vi "Register Variation.vi"() -> ()   [LabVIEW 2014]
uses:
  TypeDef/state.ctl
  TypeDef/Qmessage.ctl
  <vilib>/Utility/config.llb/Read Key (Path).vi
  <vilib>/Utility/file.llb/Read From Spreadsheet File (string).vi
  <vilib>/Utility/config.llb/Write Key (Path).vi
  <vilib>/Utility/config.llb/NI_LVConfig.lvlib
panel:
  in  "Help Button":bool
  in  "Run":bool
  in  "Initialize":bool
  out "Status bar":string
  in  "Register change":bool
  in  "Add comment":bool
  in  "View":bool
  in  "NV 31":string
  in  "NV 30":string
  in  "NV 29":string
  in  "NV 28":string
  in  "NV 27":string
  in  "NV 26":string
  in  "NV 25":string
  in  "NV 24":string
  in  "NV 23":string
  in  "NV 22":string
  in  "NV 21":string
  in  "NV 20":string
  in  "NV 19":string
  in  "NV 18":string
  in  "NV 17":string
  in  "NV 16":string
  in  "NV 15":string
  in  "NV 14":string
  in  "NV 13":string
  in  "NV 12":string
  in  "NV 11":string
  in  "NV 10":string
  in  "NV 9":string
  in  "NV 8":string
  in  "NV 7":string
  in  "NV 6":string
  in  "NV 5":string
  in  "NV 4":string
  in  "NV 3":string
  in  "NV 2":string
  in  "NV 1":string
  out "V 31":string
  out "V 30":string
  out "V 29":string
  out "V 28":string
  out "V 27":string
  out "V 26":string
  out "V 25":string
  out "V 24":string
  out "V 23":string
  out "V 22":string
  out "V 21":string
  out "V 20":string
  out "V 19":string
  out "V 18":string
  out "V 17":string
  out "V 16":string
  out "V 15":string
  out "V 14":string
  out "V 13":string
  out "V 12":string
  out "V 11":string
  out "V 10":string
  out "V 9":string
  out "V 8":string
  out "V 7":string
  out "V 6":string
  out "V 5":string
  out "V 4":string
  out "V 3":string
  out "V 2":string
  out "V 1":string
  in  "tdms path":path caption="Variation Registry (*.tdms)"
  in  "Config Path":path caption="Config Path (*.txt)"
  out "N 31":string
  out "N 30":string
  out "N 29":string
  out "N 28":string
  out "N 27":string
  out "N 26":string
  out "N 25":string
  out "N 24":string
  out "N 23":string
  out "N 22":string
  out "N 21":string
  out "N 20":string
  out "N 19":string
  out "N 18":string
  out "N 17":string
  out "N 16":string
  out "N 15":string
  out "N 14":string
  out "N 13":string
  out "N 12":string
  out "N 11":string
  out "N 10":string
  out "N 9":string
  out "N 8":string
  out "N 7":string
  out "N 6":string
  out "N 5":string
  out "N 4":string
  out "N 3":string
  out "N 2":string
  out "N 1":string
  in  "Exit":bool
  # "Change Register"
  # "Current Configuration"
  # "New Configuration"
  # "Component Name"
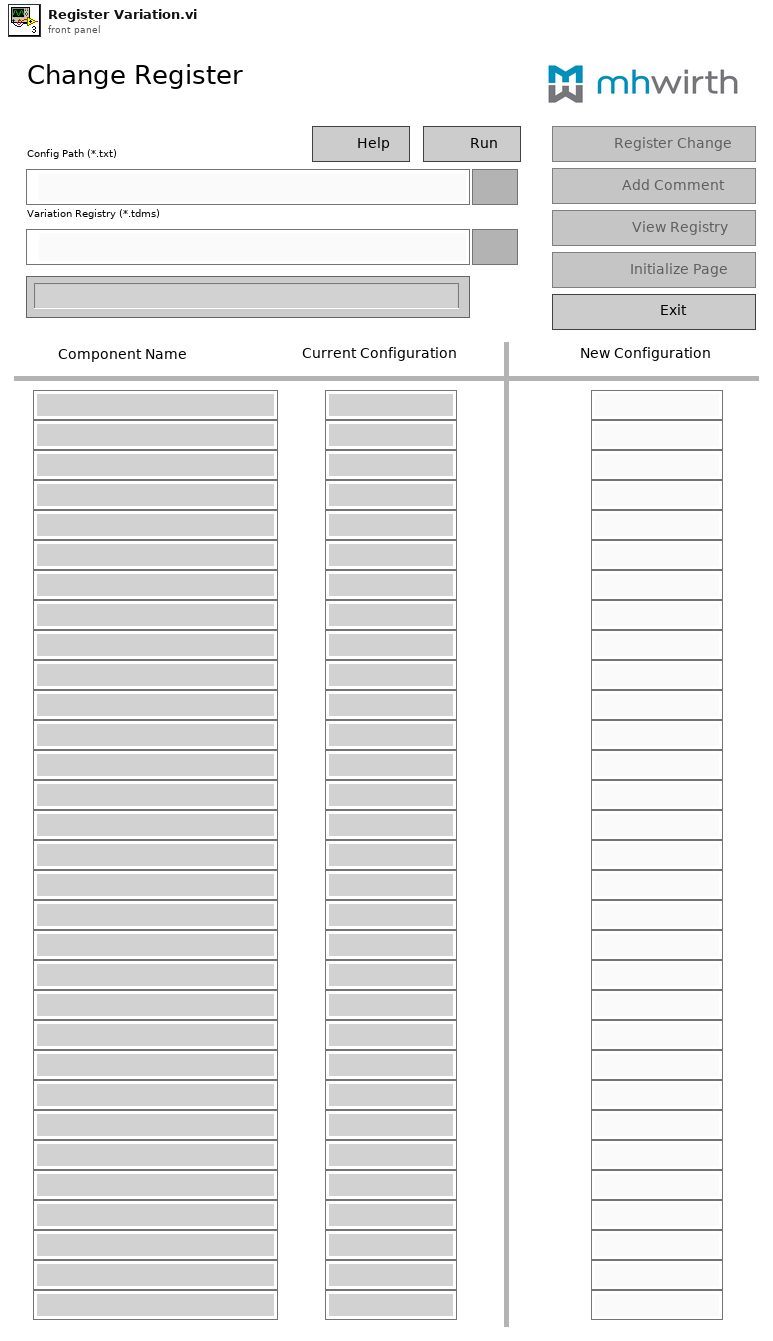
[diagram p1: front panel]
types:
  T1 = typedef "Qmessage.ctl" = cluster{"data":variant, "state":T2}
  T2 = typedef "state.ctl" = enum16{"Run", "Initialize 1", "Initialize 2", "Read config file", "Read TDMS", "Config file Error", "Idle", "Update Comp Names", "Update Current Versions", "Make new configuration", "Register Change", "View Registry", "Add Comment", "No New Update", "Check current versions", "Read ini file", "Write ini file", "Close"}
  T3 = enum32{"invalid app kind", "Development System", "Run Time System", "Student Edition", "Embedded LabVIEW", "Evaluation", "Custom"}
  T4 = cluster{"keys":refnum<vi>[], "Names":refnum<vi>[], "Current Versions":refnum<vi>[], "New Versions":refnum<vi>[]}
  T5 = enum8{"Enabled", "Disabled", "Disabled and Grayed Out"}
  T6 = typedef "NI_LVConfig.lvlib/Config Data RefNum.ctl" = refnum<k1>
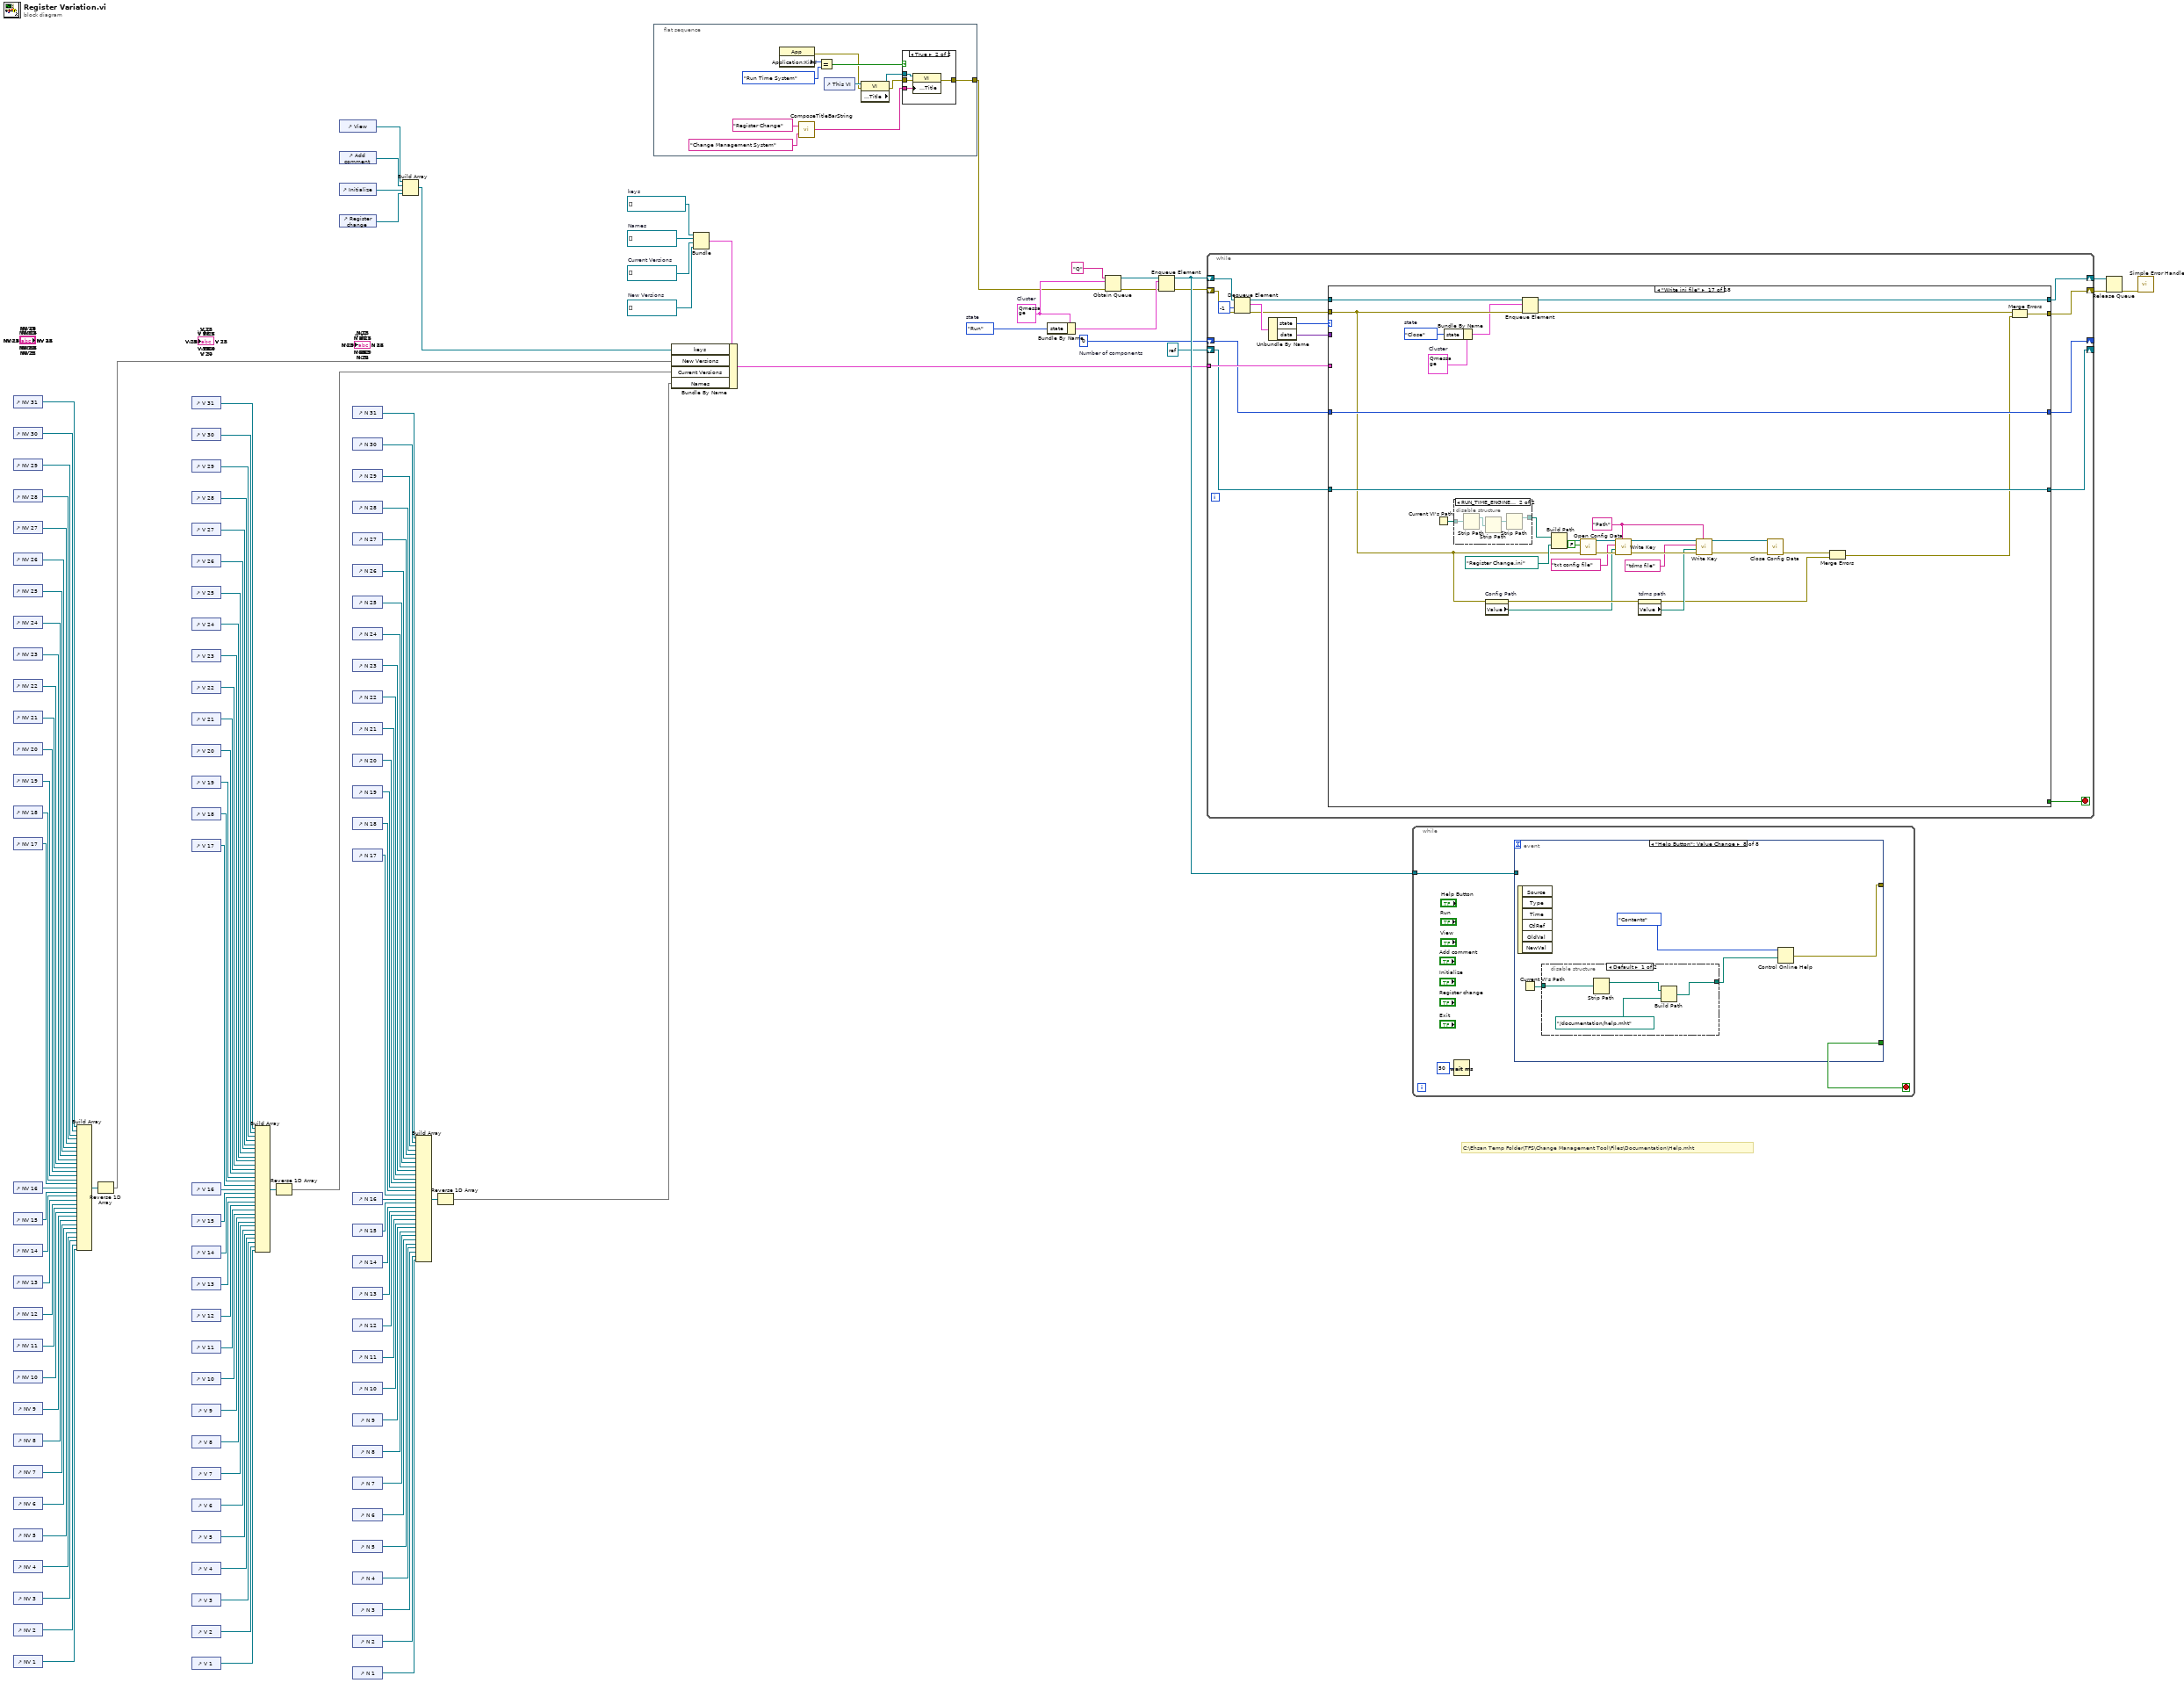
[diagram p0: block diagram]
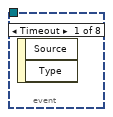
[diagram p3: hidden frame]
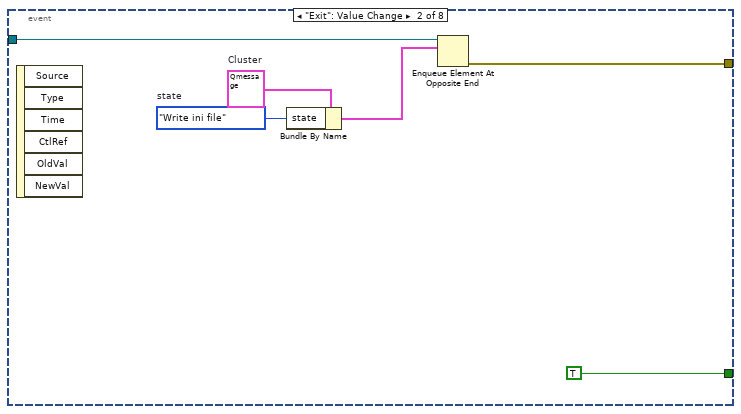
[diagram p4: hidden frame]
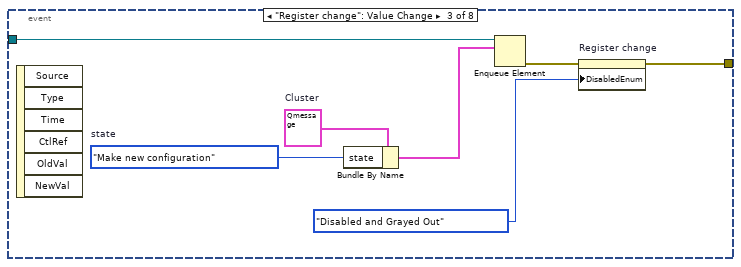
[diagram p5: hidden frame]
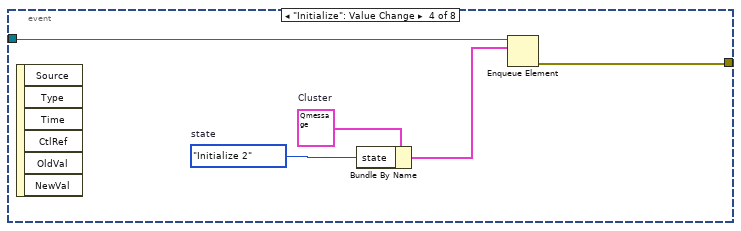
[diagram p6: hidden frame]
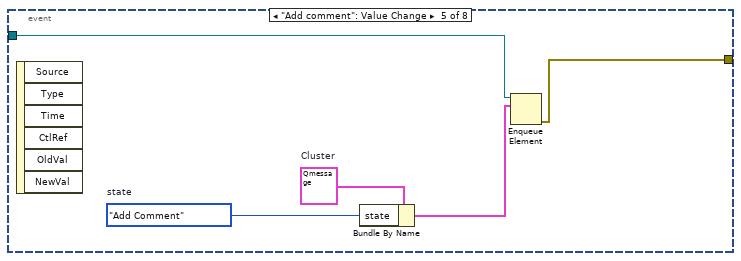
[diagram p7: hidden frame]
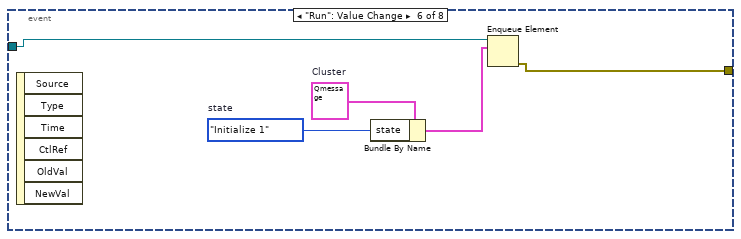
[diagram p8: hidden frame]
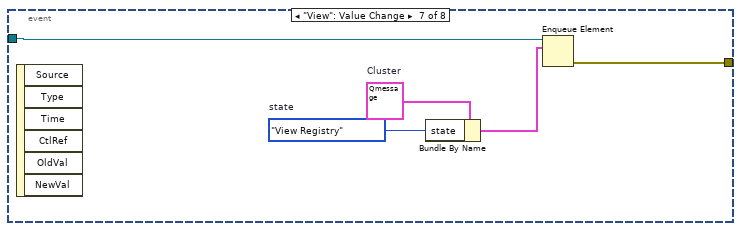
[diagram p9: hidden frame]
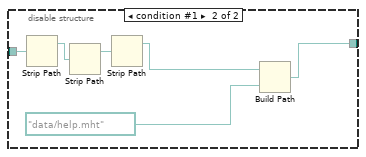
[diagram p10: hidden frame]
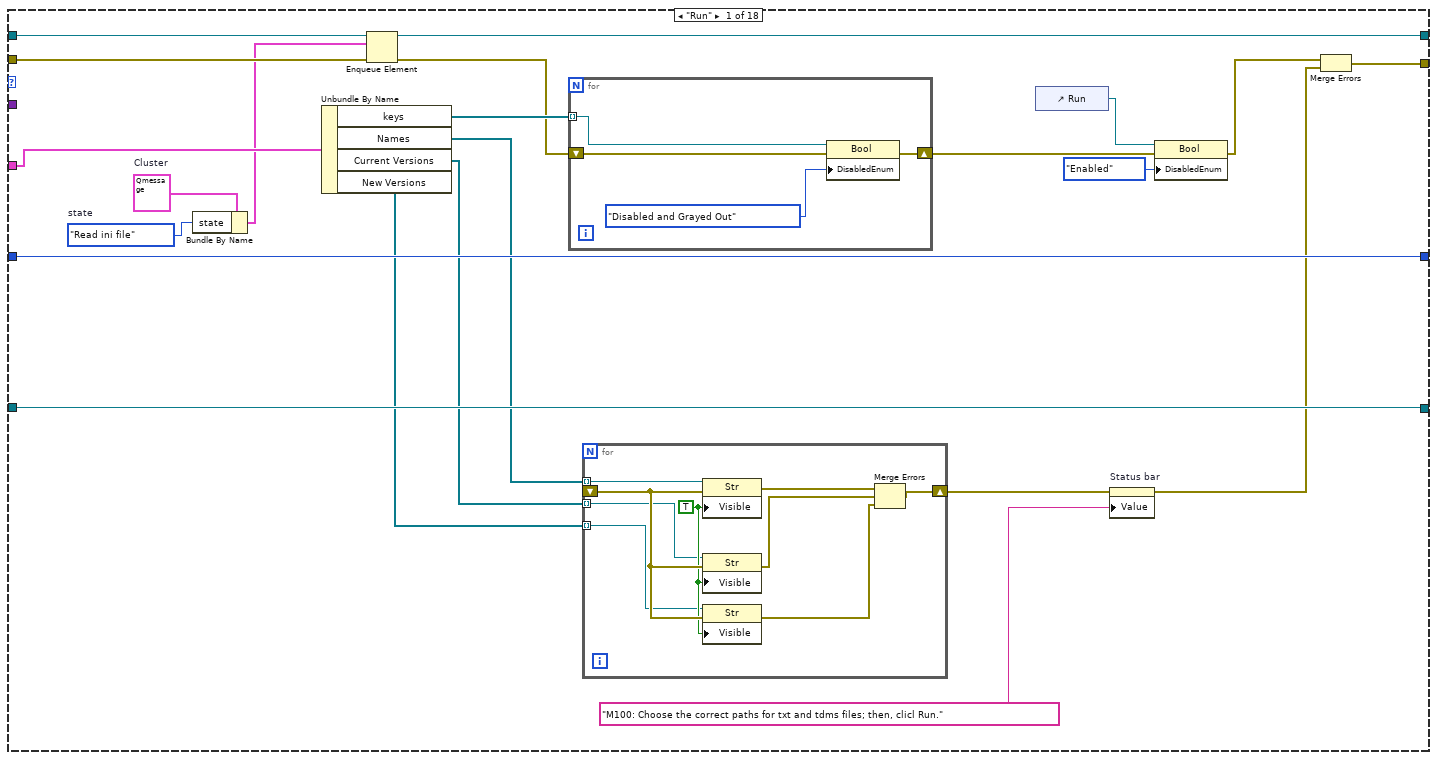
[diagram p11: hidden frame]
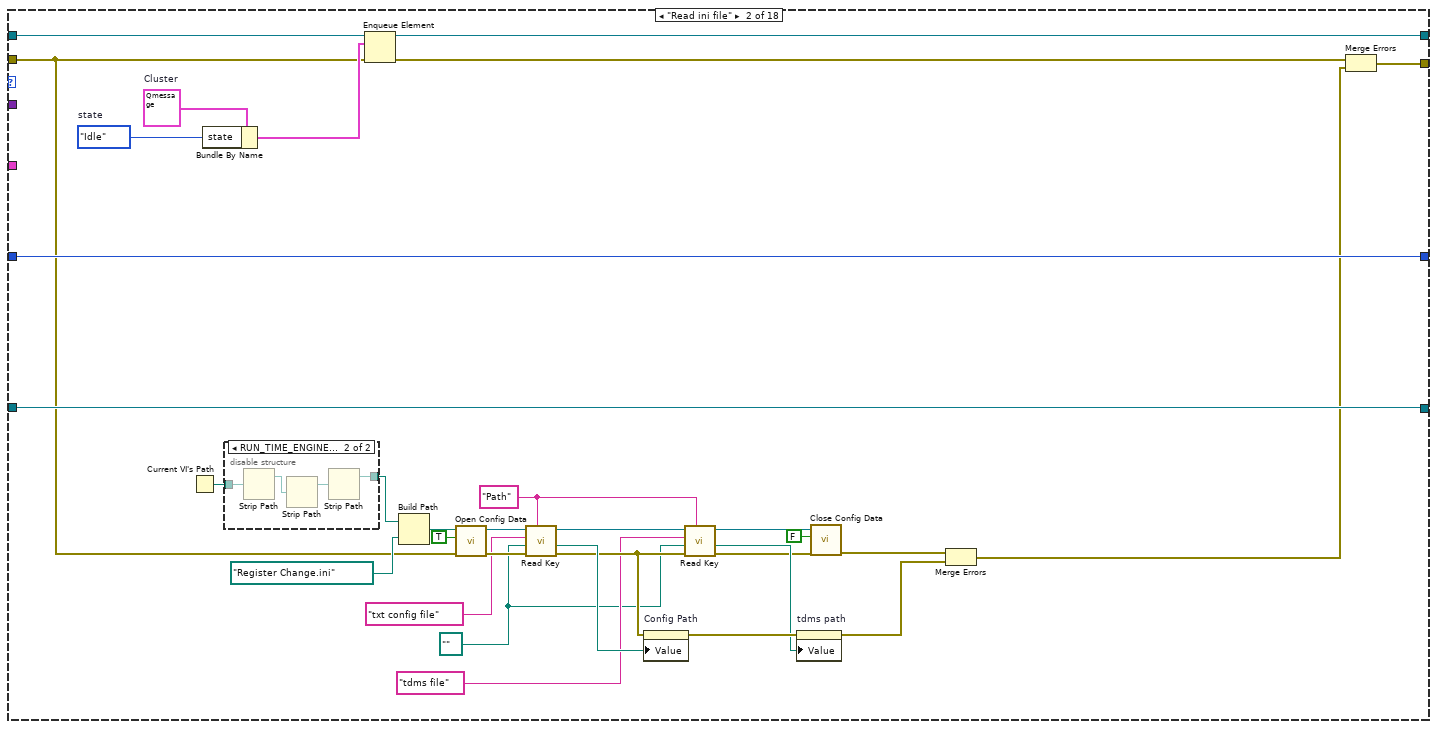
[diagram p12: hidden frame]
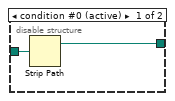
[diagram p13: hidden frame]
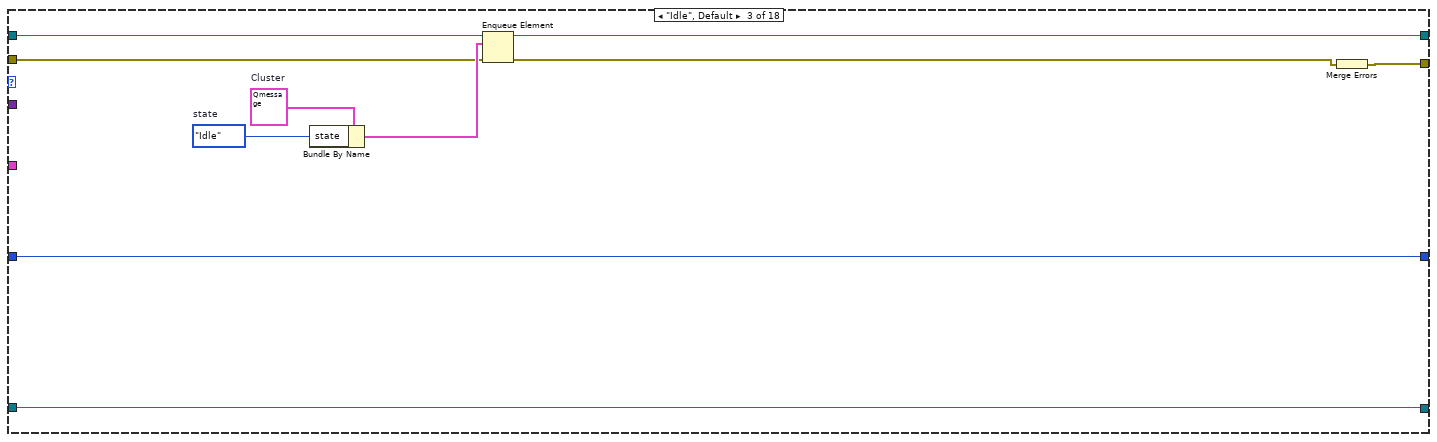
[diagram p14: hidden frame]
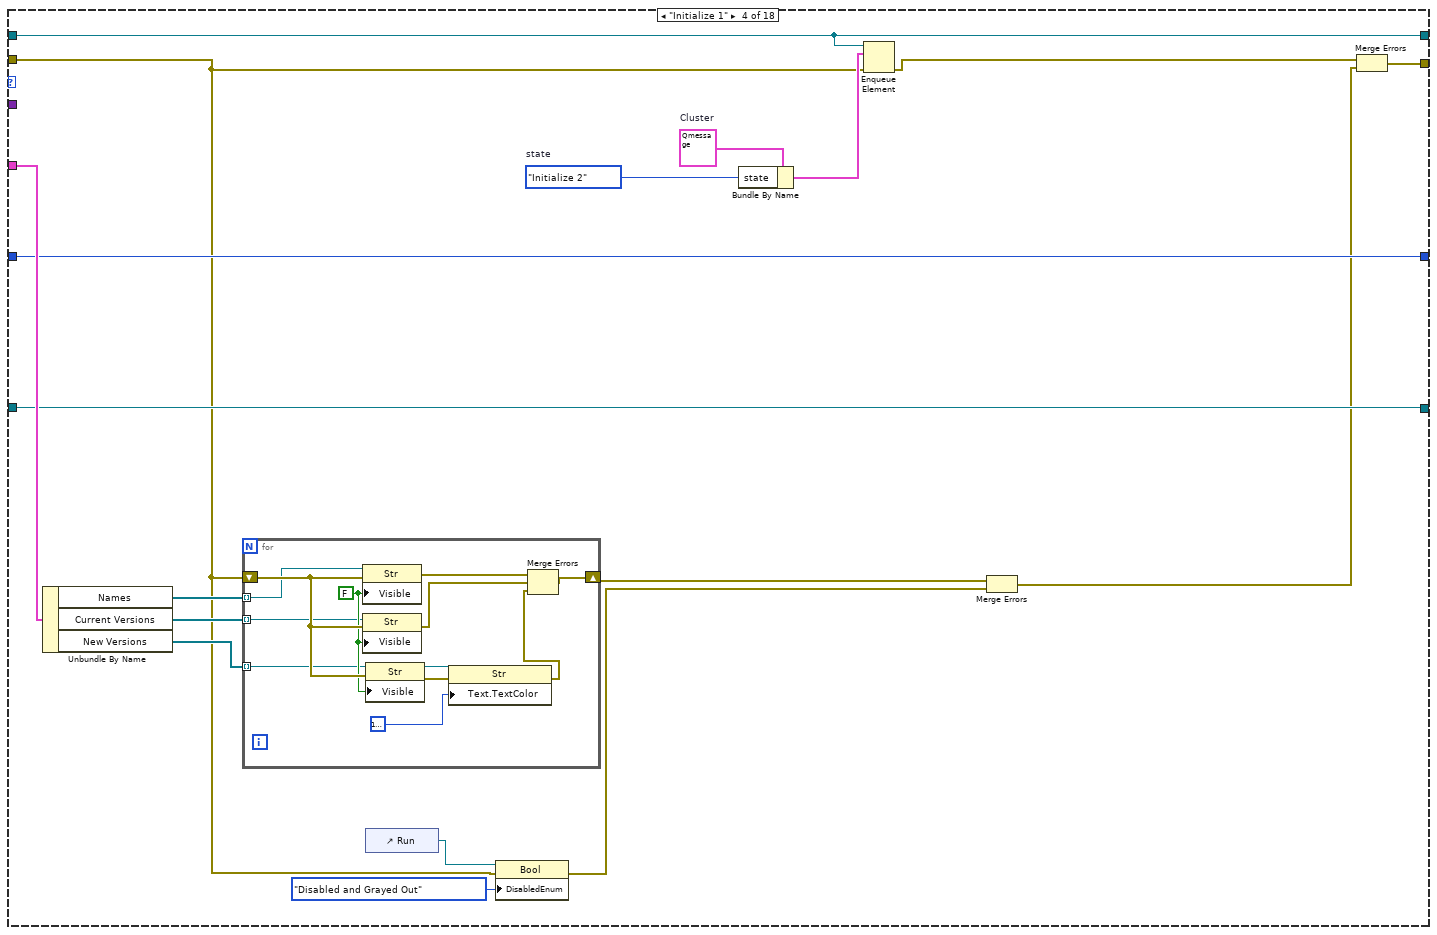
[diagram p15: hidden frame]
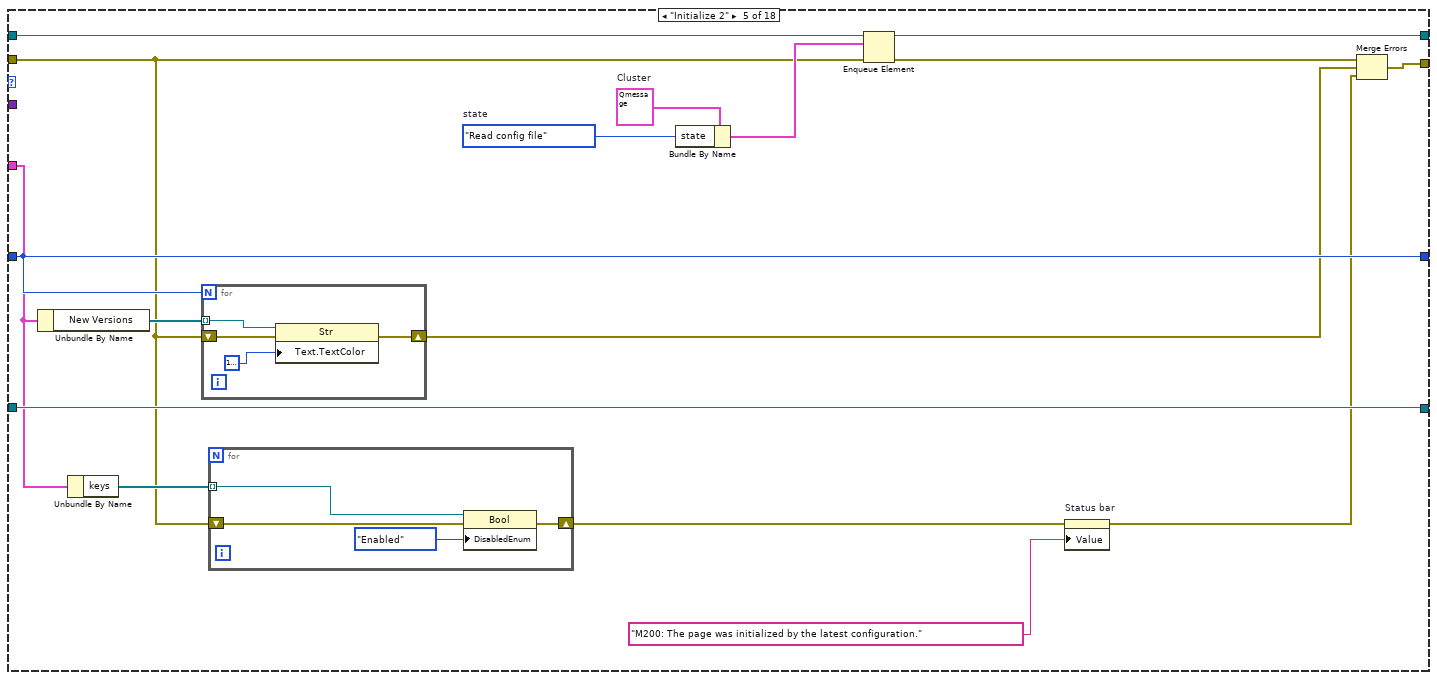
[diagram p16: hidden frame]
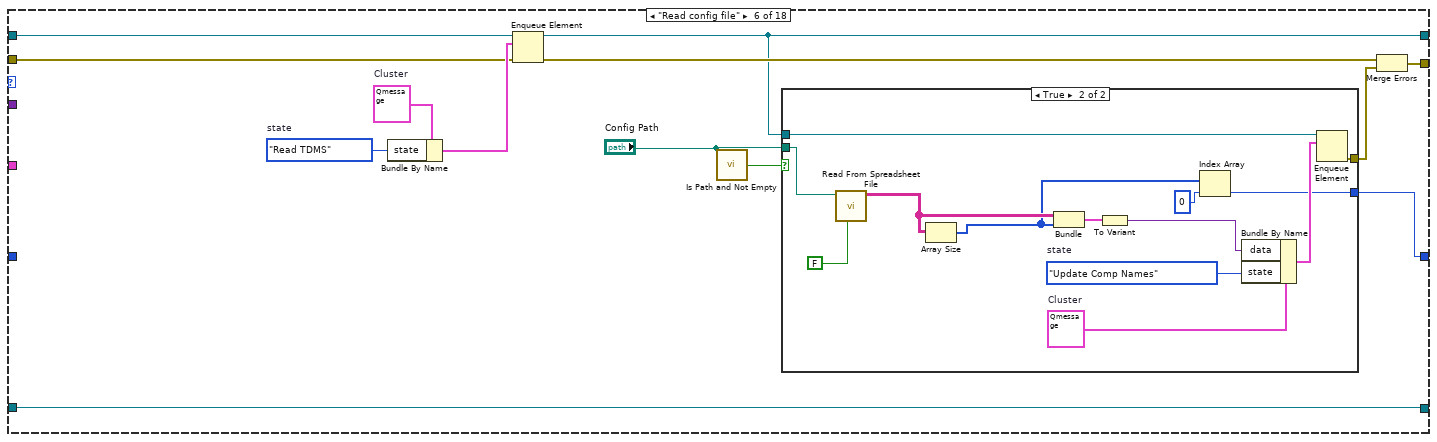
[diagram p17: hidden frame]
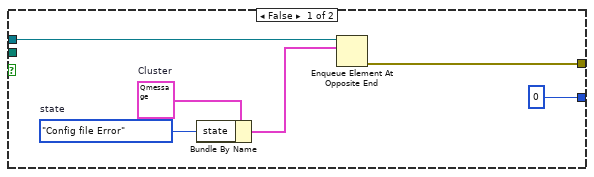
[diagram p18: hidden frame]
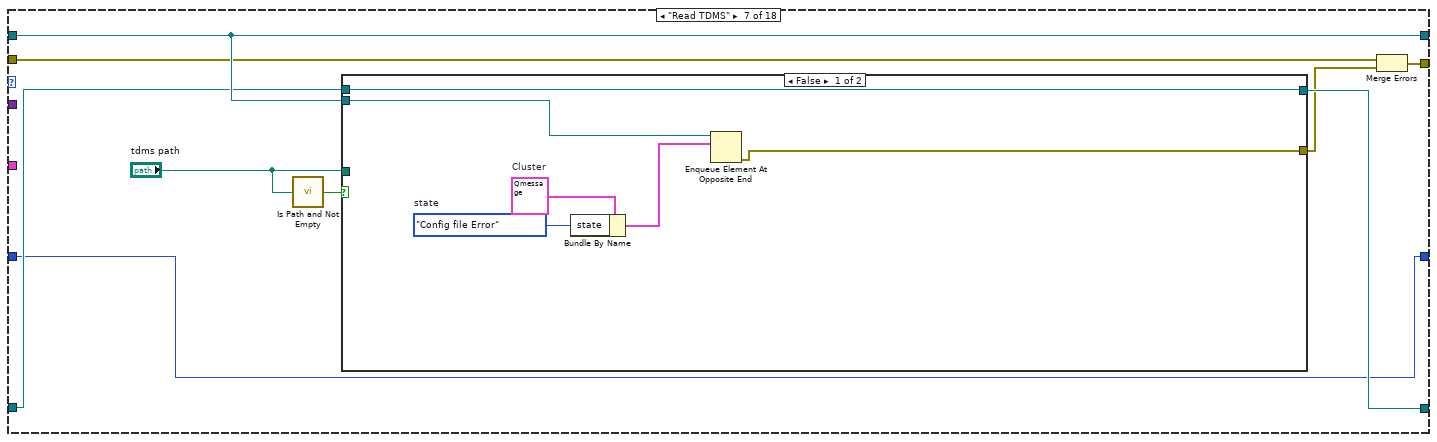
[diagram p19: hidden frame]
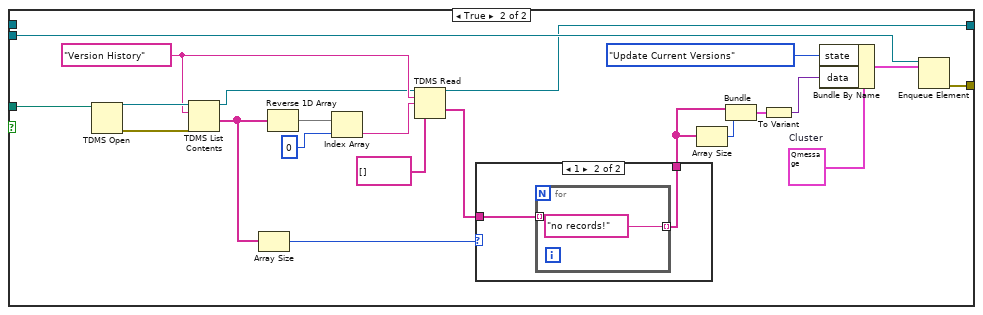
[diagram p20: hidden frame]
diagram:
  w15 = refnum<vi>[] []  # keys
  w21 = 0  # Number of components
  w12 = refnum<vi>[] []  # New Versions
  w13 = refnum<vi>[] []  # Current Versions
  w14 = refnum<vi>[] []  # Names
  w121 = T1 {"data"=variant, "state"=enum."Initialize 1"}  # Cluster
  w124 = state."Run"  # state
  # "C:\\Ehsan Temp Folder\\TFS\\Change Management Tool\\Files\\Documentation\\Help.mht"
  n1 = control-ref of="NV 31"() -> (w54:refnum<vi>)
  n2 = control-ref of="NV 30"() -> (w53:refnum<vi>)
  n3 = control-ref of="NV 29"() -> (w52:refnum<vi>)
  n4 = control-ref of="NV 28"() -> (w51:refnum<vi>)
  n5 = control-ref of="NV 27"() -> (w50:refnum<vi>)
  n6 = control-ref of="NV 26"() -> (w49:refnum<vi>)
  n7 = control-ref of="NV 25"() -> (w48:refnum<vi>)
  n8 = control-ref of="NV 24"() -> (w47:refnum<vi>)
  n9 = control-ref of="NV 23"() -> (w46:refnum<vi>)
  n10 = control-ref of="NV 22"() -> (w45:refnum<vi>)
  n11 = control-ref of="NV 21"() -> (w44:refnum<vi>)
  n12 = control-ref of="NV 20"() -> (w43:refnum<vi>)
  n13 = control-ref of="NV 19"() -> (w42:refnum<vi>)
  n14 = control-ref of="NV 18"() -> (w41:refnum<vi>)
  n15 = control-ref of="NV 17"() -> (w40:refnum<vi>)
  n16 = control-ref of="NV 16"() -> (w39:refnum<vi>)
  n17 = control-ref of="NV 15"() -> (w38:refnum<vi>)
  n18 = control-ref of="NV 14"() -> (w37:refnum<vi>)
  n19 = control-ref of="NV 13"() -> (w36:refnum<vi>)
  n20 = control-ref of="NV 12"() -> (w35:refnum<vi>)
  n21 = control-ref of="NV 11"() -> (w34:refnum<vi>)
  n22 = control-ref of="NV 10"() -> (w33:refnum<vi>)
  n23 = control-ref of="NV 9"() -> (w32:refnum<vi>)
  n24 = control-ref of="NV 8"() -> (w31:refnum<vi>)
  n25 = control-ref of="NV 7"() -> (w30:refnum<vi>)
  n26 = control-ref of="NV 6"() -> (w29:refnum<vi>)
  n27 = control-ref of="NV 5"() -> (w28:refnum<vi>)
  n28 = control-ref of="NV 4"() -> (w27:refnum<vi>)
  n29 = control-ref of="NV 3"() -> (w26:refnum<vi>)
  n30 = control-ref of="NV 2"() -> (w25:refnum<vi>)
  n31 = control-ref of="NV 1"() -> (w24:refnum<vi>)
  n32 = Build Array(w54, w53, w52, w51, w50, w49, w48, w47, w46, w45, w44, w43, w42, w41, w40, w39, w38, w37, w36, w35, w34, w33, w32, w31, w30, w29, w28, w27, w26, w25, w24) -> (w23:refnum<vi>[])
  n33 = Reverse 1D Array(array=w23) -> (reversed array=w6:refnum<vi>[])
  n34 = control-ref of="V 31"() -> (w86:refnum<vi>)
  n35 = control-ref of="V 30"() -> (w85:refnum<vi>)
  n36 = control-ref of="V 29"() -> (w84:refnum<vi>)
  n37 = control-ref of="V 28"() -> (w83:refnum<vi>)
  n38 = control-ref of="V 27"() -> (w82:refnum<vi>)
  n39 = control-ref of="V 26"() -> (w81:refnum<vi>)
  n40 = control-ref of="V 25"() -> (w80:refnum<vi>)
  n41 = control-ref of="V 24"() -> (w79:refnum<vi>)
  n42 = control-ref of="V 23"() -> (w78:refnum<vi>)
  n43 = control-ref of="V 22"() -> (w77:refnum<vi>)
  n44 = control-ref of="V 21"() -> (w76:refnum<vi>)
  n45 = control-ref of="V 20"() -> (w75:refnum<vi>)
  n46 = control-ref of="V 19"() -> (w74:refnum<vi>)
  n47 = control-ref of="V 18"() -> (w73:refnum<vi>)
  n48 = control-ref of="V 17"() -> (w72:refnum<vi>)
  n49 = control-ref of="V 16"() -> (w71:refnum<vi>)
  n50 = control-ref of="V 15"() -> (w70:refnum<vi>)
  n51 = control-ref of="V 14"() -> (w69:refnum<vi>)
  n52 = control-ref of="V 13"() -> (w68:refnum<vi>)
  n53 = control-ref of="V 12"() -> (w67:refnum<vi>)
  n54 = control-ref of="V 11"() -> (w66:refnum<vi>)
  n55 = control-ref of="V 10"() -> (w65:refnum<vi>)
  n56 = control-ref of="V 9"() -> (w64:refnum<vi>)
  n57 = control-ref of="V 8"() -> (w63:refnum<vi>)
  n58 = control-ref of="V 7"() -> (w62:refnum<vi>)
  n59 = control-ref of="V 6"() -> (w61:refnum<vi>)
  n60 = control-ref of="V 5"() -> (w60:refnum<vi>)
  n61 = control-ref of="V 4"() -> (w59:refnum<vi>)
  n62 = control-ref of="V 3"() -> (w58:refnum<vi>)
  n63 = control-ref of="V 2"() -> (w57:refnum<vi>)
  n64 = control-ref of="V 1"() -> (w56:refnum<vi>)
  n65 = Build Array(w86, w85, w84, w83, w82, w81, w80, w79, w78, w77, w76, w75, w74, w73, w72, w71, w70, w69, w68, w67, w66, w65, w64, w63, w62, w61, w60, w59, w58, w57, w56) -> (w55:refnum<vi>[])
  n66 = Reverse 1D Array(array=w55) -> (reversed array=w7:refnum<vi>[])
  n67 = control-ref of="View"() -> (w20:refnum<vi>)
  n68 = control-ref of="Add comment"() -> (w19:refnum<vi>)
  n69 = control-ref of="Initialize"() -> (w18:refnum<vi>)
  n70 = control-ref of="Register change"() -> (w17:refnum<vi>)
  n71 = control-ref of="N 31"() -> (w119:refnum<vi>)
  n72 = control-ref of="N 30"() -> (w118:refnum<vi>)
  n73 = control-ref of="N 29"() -> (w117:refnum<vi>)
  n74 = control-ref of="N 28"() -> (w116:refnum<vi>)
  n75 = control-ref of="N 27"() -> (w115:refnum<vi>)
  n76 = control-ref of="N 26"() -> (w114:refnum<vi>)
  n77 = control-ref of="N 25"() -> (w113:refnum<vi>)
  n78 = control-ref of="N 24"() -> (w112:refnum<vi>)
  n79 = control-ref of="N 23"() -> (w111:refnum<vi>)
  n80 = control-ref of="N 22"() -> (w110:refnum<vi>)
  n81 = control-ref of="N 21"() -> (w109:refnum<vi>)
  n82 = control-ref of="N 20"() -> (w108:refnum<vi>)
  n83 = control-ref of="N 19"() -> (w107:refnum<vi>)
  n84 = control-ref of="N 18"() -> (w106:refnum<vi>)
  n85 = control-ref of="N 17"() -> (w105:refnum<vi>)
  n86 = control-ref of="N 16"() -> (w104:refnum<vi>)
  n87 = control-ref of="N 15"() -> (w103:refnum<vi>)
  n88 = control-ref of="N 14"() -> (w102:refnum<vi>)
  n89 = control-ref of="N 13"() -> (w101:refnum<vi>)
  n90 = control-ref of="N 12"() -> (w100:refnum<vi>)
  n91 = control-ref of="N 11"() -> (w99:refnum<vi>)
  n92 = control-ref of="N 10"() -> (w98:refnum<vi>)
  n93 = control-ref of="N 9"() -> (w97:refnum<vi>)
  n94 = control-ref of="N 8"() -> (w96:refnum<vi>)
  n95 = control-ref of="N 7"() -> (w95:refnum<vi>)
  n96 = control-ref of="N 6"() -> (w94:refnum<vi>)
  n97 = control-ref of="N 5"() -> (w93:refnum<vi>)
  n98 = control-ref of="N 4"() -> (w92:refnum<vi>)
  n99 = control-ref of="N 3"() -> (w91:refnum<vi>)
  n100 = control-ref of="N 2"() -> (w90:refnum<vi>)
  n101 = control-ref of="N 1"() -> (w89:refnum<vi>)
  n102 = Build Array(w20, w19, w18, w17) -> (w9:refnum<vi>[])
  n103 = Build Array(w119, w118, w117, w116, w115, w114, w113, w112, w111, w110, w109, w108, w107, w106, w105, w104, w103, w102, w101, w100, w99, w98, w97, w96, w95, w94, w93, w92, w91, w90, w89) -> (w88:refnum<vi>[])
  n104 = Reverse 1D Array(array=w88) -> (reversed array=w8:refnum<vi>[])
  n105 = flat-sequence {
    tunnel: [w125] -> w16
    frame #0 {
      n106 = property on="Property Node" class="App"() -> (error out=w127:errorcluster, "Application:Kind"=w133:T3)  [unwired: 2 in, 1 out]
      n107 = call "ComposeTitleBarString.vi"("ProjectName"="Change Management System" ("Application"), "Application"="Register Change") -> ("TitleBar"=w135:string)
      n108 = Equal?(x=w133, y=T3."Run Time System" ("Applikation:Typ")) -> (x = y?=w134:bool)
      n109 = control-ref of="This VI"() -> (w131:refnum<vi>)
      n110 = property on="Property Node" class="VI" props=["Front Panel.Title"](reference=w131, error in=w127) -> (reference out=w130:refnum<vi>, error out=w126:errorcluster)  [unwired: 1 out]
      n111 = case shown="True" w134 {
        tunnel: w135 -> [_ w140]
        tunnel: w130 -> [_ w139]
        tunnel: w126 -> [w136 w138]
        tunnel: [w136 w137] -> w125
        frame False {
        }
        frame True {
          n112 = property class="VI"(reference=w139, error in=w138, "Front Panel.Title"=w140) -> (error out=w137:errorcluster)  [unwired: 1 out]
        }
      }
    }
  }
  n113 = Bundle("keys"=w15, "Names"=w14, "Current Versions"=w13, "New Versions"=w12) -> (w10:T4)  [unwired: 1 in]
  n114 = Bundle By Name(cluster=w10, "keys"=w9, "New Versions"=w6, "Current Versions"=w7, "Names"=w8) -> (w11:T4)
  n115 = Bundle By Name(cluster=w121, "state"=w124) -> (w120:T1)
  n116 = Obtain Queue(name (unnamed)="Q", element data type=w121, error in (no error)=w16) -> (queue out=w123:refnum<queue>, error out=w5:errorcluster)  [unwired: 2 in, 1 out]
  n117 = Enqueue Element(queue=w123, element=w120, error in (no error)=w5) -> (queue out=w87:refnum<queue>, error out=w4:errorcluster)  [unwired: 1 in, 1 out]
  n118 = while {
    shift-right: [w150] -> w2
    shift-left: w87 -> [w154]
    shift-right: [w149] -> w3
    shift-left: w4 -> [w156]
    tunnel: w11 -> [w145]
    shift-right: [w144] -> _
    shift-left: refnum<k34> refnum ("tdms file out") -> [w143]
    shift-right: [w142] -> _
    shift-left: w21 -> [w141]
    stop <- w146 stop-if-true
    n119 = Dequeue Element(queue=w154, timeout in ms (-1)=-1, error in (no error)=w156) -> (queue out=w151:refnum<queue>, element=w155:T1, error out=w147:errorcluster)  [unwired: 1 out]
    n120 = Unbundle By Name(w155) -> ("state"=w153:T2, "data"=w152:variant)
    n121 = case shown="\"Write ini file\"" w153 {
      tunnel: w152 -> [_ _ _ _ _ _ _ w384 w407 _ w491 _ _ _ _ _ _ _]
      tunnel: w151 -> [w161 w221 w235 w249 w279 w297 w333 w376 w400 w434 w485 w520 w548 w563 w579 w591 w609 w652]
      tunnel: [w160 w220 w234 w249 w278 w296 w333 w376 w400 w434 w485 w520 w548 w563 w579 w591 w608 w652] -> w150
      tunnel: w147 -> [w159 w214 w232 w242 w272 w299 w332 w381 w404 w443 w490 w525 w532 w566 w574 w597 w607 w642]
      tunnel: [w171 w200 w231 w252 w285 w307 w335 w375 w399 w436 w486 w517 w528 w562 w573 w597 w612 w649] -> w149
      tunnel: [_ _ _ _ _ _ _ _ _ _ _ _ _ _ _ _ _ TRUE] -> w146
      tunnel: w145 -> [w176 _ _ w257 w273 _ _ w371 w398 w446 _ _ _ _ w576 _ _ _]
      tunnel: [w178 w223 w239 w246 w280 w303 w331 w369 w395 w447 w487 w526 w538 w568 w578 w593 w631 w645] -> w144
      tunnel: w143 -> [w178 w223 w239 w246 w280 w303 w330 w369 w395 w447 w487 w526 w542 w568 w578 w593 w631 w645]
      tunnel: [w177 w222 w238 w253 w274 w295 w329 w368 w393 w440 w479 w527 w547 w567 w577 w592 w630 w647] -> w142
      tunnel: w141 -> [w177 w222 w238 w253 w274 _ w329 w368 w393 w440 w479 w527 w547 w567 w577 w592 w630 w647]
      frame "Run" {
        w163 = T1 {"data"=variant, "state"=enum."Initialize 1"}  # Cluster
        w162 = state."Read ini file"  # state
        n122 = Bundle By Name(cluster=w163, "state"=w162) -> (w157:T1)
        n123 = Unbundle By Name(w176) -> ("keys"=w175:refnum<vi>[], "Names"=w174:refnum<vi>[], "Current Versions"=w173:refnum<vi>[], "New Versions"=w172:refnum<vi>[])
        n124 = Enqueue Element(queue=w161, element=w157, error in (no error)=w159) -> (queue out=w160:refnum<queue>, error out=w158:errorcluster)  [unwired: 1 in, 1 out]
        n125 = for {
          shift-right: [w189] -> w168
          shift-left: w158 -> [w190]
          tunnel: w175 -> [w188] mode=indexing
          n126 = property class="Bool"(reference=w188, error in=w190, "DisabledEnum"=T5."Disabled and Grayed Out" ("Disabled")) -> (error out=w189:errorcluster)  [unwired: 1 out]
        }
        n127 = for {
          shift-right: [w187] -> w166
          shift-left: _ -> [w184]
          tunnel: w174 -> [w181] mode=indexing
          tunnel: w173 -> [w180] mode=indexing
          tunnel: w172 -> [w179] mode=indexing
          w183 = TRUE ("Visible")
          n128 = property class="Str"(reference=w181, error in=w184, "Visible"=w183) -> (error out=w186:errorcluster)  [unwired: 1 out]
          n129 = property class="Str"(reference=w180, error in=w184, "Visible"=w183) -> (error out=w185:errorcluster)  [unwired: 1 out]
          n130 = property class="Str"(reference=w179, error in=w184, "Visible"=w183) -> (error out=w182:errorcluster)  [unwired: 1 out]
          n131 = Merge Errors(w186, w185, w182) -> (w187:errorcluster)
        }
        n132 = control-ref of="Run"() -> (w170:refnum<vi>)
        n133 = property on="Status bar" class="Str"(error in=w166, "Value"="M100: Choose the correct paths for txt and tdms files; then, clicl Run." ("Status bar")) -> (error out=w165:errorcluster)  [unwired: 1 in, 1 out]
        n134 = property class="Bool"(reference=w170, error in=w168, "DisabledEnum"=T5."Enabled" ("Disabled")) -> (error out=w167:errorcluster)  [unwired: 1 out]
        n135 = Merge Errors(w167, w165) -> (w171:errorcluster)
      }
      frame "Read ini file" {
        w206 = path "" ("default value")
        w205 = "Path" ("section")
        w219 = T1 {"data"=variant, "state"=enum."Initialize 1"}  # Cluster
        w218 = state."Idle"  # state
        n136 = Current VI's Path() -> (path=w193:path)
        n137 = Bundle By Name(cluster=w219, "state"=w218) -> (w217:T1)
        n138 = disable-structure shown="RUN_TIME_ENGINE==True" {
          disable-tunnel: w193 -> [w225 w229]
          disable-tunnel: [w224 w226] -> w192
          frame condition #0 (active) {
            n139 = Strip Path(path=w225) -> (stripped path=w224:path)  [unwired: 1 out]
          }
          frame condition #1 {
            n140 = Strip Path(path=w229) -> (stripped path=w228:path)  [unwired: 1 out]
            n141 = Strip Path(path=w228) -> (stripped path=w227:path)  [unwired: 1 out]
            n142 = Strip Path(path=w227) -> (stripped path=w226:path)  [unwired: 1 out]
          }
        }
        n143 = Enqueue Element(queue=w221, element=w217, error in (no error)=w214) -> (queue out=w220:refnum<queue>, error out=w201:errorcluster)  [unwired: 1 in, 1 out]
        n144 = Build Path(base path=w192, name or relative path=path "Register Change.ini") -> (appended path=w215:path)
        n145 = call <vilib>:"Open Config Data.vi"("error in (no error)"=w214, "create file if necessary (T)"=TRUE, "configuration file path"=w215) -> ("error out"=w212:errorcluster, "refnum"=w213:T6)  [unwired: 6 in, 1 out]
        n146 = call-poly <vilib>:"Read Key.vi"("section"=w205, "error in (no error)"=w212, "default value"=w206, "key"="txt config file", "refnum"=w213) -> ("error out"=w209:errorcluster, "value"=w210:path, "refnum out"=w208:T6)  [unwired: 3 in, 1 out]
        n147 = property on="Config Path" class="Path"(error in=w209, "Value"=w210) -> (error out=w204:errorcluster)  [unwired: 1 in, 1 out]
        n148 = call-poly <vilib>:"Read Key.vi"("section"=w205, "error in (no error)"=w209, "default value"=w206, "key"="tdms file", "refnum"=w208) -> ("error out"=w197:errorcluster, "value"=w203:path, "refnum out"=w198:T6)  [unwired: 3 in, 1 out]
        n149 = property on="tdms path" class="Path"(error in=w204, "Value"=w203) -> (error out=w199:errorcluster)  [unwired: 1 in, 1 out]
        n150 = call <vilib>:"Close Config Data.vi"("error in (no error)"=w197, "write file if changed (T)"=FALSE, "refnum"=w198) -> ("error out"=w195:errorcluster)  [unwired: 8 out]
        n151 = Merge Errors(w195, w199) -> (w202:errorcluster)
        n152 = Merge Errors(w201, w202) -> (w200:errorcluster)
      }
      frame "Idle", Default {
        w237 = T1 {"data"=variant, "state"=enum."Initialize 1"}  # Cluster
        w236 = state."Idle"  # state
        n153 = Bundle By Name(cluster=w237, "state"=w236) -> (w233:T1)
        n154 = Enqueue Element(queue=w235, element=w233, error in (no error)=w232) -> (queue out=w234:refnum<queue>, error out=w230:errorcluster)  [unwired: 1 in, 1 out]
        n155 = Merge Errors(w230) -> (w231:errorcluster)
      }
      frame "Initialize 1" {
        w251 = T1 {"data"=variant, "state"=enum."Initialize 1"}  # Cluster
        w250 = state."Initialize 2"  # state
        n156 = Unbundle By Name(w257) -> ("Names"=w256:refnum<vi>[], "Current Versions"=w255:refnum<vi>[], "New Versions"=w254:refnum<vi>[])
        n157 = for {
          shift-right: [w269] -> w245
          shift-left: w242 -> [w266]
          tunnel: w256 -> [w264] mode=indexing
          tunnel: w255 -> [w263] mode=indexing
          tunnel: w254 -> [w262] mode=indexing
          w265 = FALSE ("Visible")
          n158 = property class="Str"(reference=w264, error in=w266, "Visible"=w265) -> (error out=w268:errorcluster)  [unwired: 1 out]
          n159 = property class="Str"(reference=w263, error in=w266, "Visible"=w265) -> (error out=w267:errorcluster)  [unwired: 1 out]
          n160 = property class="Str"(reference=w262, error in=w266, "Visible"=w265) -> (reference out=w260:refnum<vi>, error out=w259:errorcluster)
          n161 = property class="Str"(reference=w260, error in=w259, "Text.TextColor"=u32 16777222) -> (error out=w258:errorcluster)  [unwired: 1 out]
          n162 = Merge Errors(w268, w267, w258) -> (w269:errorcluster)
        }
        n163 = control-ref of="Run"() -> (w241:refnum<vi>)
        n164 = property class="Bool"(reference=w241, error in=w242, "DisabledEnum"=T5."Disabled and Grayed Out" ("Disabled")) -> (error out=w240:errorcluster)  [unwired: 1 out]
        n165 = Bundle By Name(cluster=w251, "state"=w250) -> (w248:T1)
        n166 = Enqueue Element(queue=w249, element=w248, error in (no error)=w242) -> (error out=w247:errorcluster)  [unwired: 1 in, 2 out]
        n167 = Merge Errors(w245, w240) -> (w244:errorcluster)
        n168 = Merge Errors(w247, w244) -> (w252:errorcluster)
      }
      frame "Initialize 2" {
        w284 = T1 {"data"=variant, "state"=enum."Initialize 1"}  # Cluster
        w283 = state."Read config file"  # state
        n169 = Unbundle By Name(w273) -> ("New Versions"=w275:refnum<vi>[])
        n170 = Unbundle By Name(w273) -> ("keys"=w277:refnum<vi>[])
        n171 = for {
          N: w274 -> [_]
          tunnel: w275 -> [w290] mode=indexing
          shift-right: [w288] -> w270
          shift-left: w272 -> [w289]
          n172 = property class="Str"(reference=w290, error in=w289, "Text.TextColor"=u32 16777222) -> (error out=w288:errorcluster)  [unwired: 1 out]
        }
        n173 = for {
          tunnel: w277 -> [w294] mode=indexing
          shift-right: [w291] -> w276
          shift-left: w272 -> [w292]
          n174 = property class="Bool"(reference=w294, error in=w292, "DisabledEnum"=T5."Enabled" ("Disabled")) -> (error out=w291:errorcluster)  [unwired: 1 out]
        }
        n175 = Bundle By Name(cluster=w284, "state"=w283) -> (w282:T1)
        n176 = Enqueue Element(queue=w279, element=w282, error in (no error)=w272) -> (queue out=w278:refnum<queue>, error out=w281:errorcluster)  [unwired: 1 in, 1 out]
        n177 = property on="Status bar" class="Str"(error in=w276, "Value"="M200: The page was initialized by the latest configuration." ("Status bar")) -> (error out=w271:errorcluster)  [unwired: 1 in, 1 out]
        n178 = Merge Errors(w281, w270, w271) -> (w285:errorcluster)
      }
      frame "Read config file" {
        w302 = T1 {"data"=variant, "state"=enum."Initialize 1"}  # Cluster
        w301 = state."Read TDMS"  # state
        n179 = Bundle By Name(cluster=w302, "state"=w301) -> (w300:T1)
        n180 = Enqueue Element(queue=w297, element=w300, error in (no error)=w299) -> (queue out=w296:refnum<queue>, error out=w298:errorcluster)  [unwired: 1 in, 1 out]
        n181 = call <vilib>:"Is Path and Not Empty.vi"("path"="Config Path") -> ("Is Path and Not Empty?"=w306:bool)  [unwired: 4 in]
        n182 = case shown="True" w306 {
          tunnel: w296 -> [w313 w320]
          tunnel: "Config Path" -> [_ w326]
          tunnel: [w309 w318] -> w305
          tunnel: [0 w314] -> w295
          frame False {
            w312 = T1 {"data"=variant, "state"=enum."Initialize 1"}  # Cluster
            w311 = state."Config file Error"  # state
            n183 = Bundle By Name(cluster=w312, "state"=w311) -> (w310:T1)
            n184 = Enqueue Element At Opposite End(queue=w313, element=w310) -> (error out=w309:errorcluster)  [unwired: 2 in, 2 out]
          }
          frame True {
            w317 = state."Update Comp Names"  # state
            w322 = T1 {"data"=variant, "state"=enum."Initialize 1"}  # Cluster
            n185 = call-poly <vilib>:"Read From Spreadsheet File.vi"("transpose (no:F)"=FALSE, "file path (dialog if empty)"=w326) -> ("all rows"=w324:string[][])  [unwired: 5 in, 4 out]
            n186 = Array Size(array=w324) -> (size(s)=w315:i32[])
            n187 = Bundle("all rows"=w324, w315) -> (w323:cluster{"all rows":string[][], i32[]})  [unwired: 1 in]
            n188 = To Variant(anything=w323) -> (Variant=w321:variant)
            n189 = Index Array(array=w315, index=0) -> (element=w314:i32)
            n190 = Bundle By Name(cluster=w322, "data"=w321, "state"=w317) -> (w319:T1)
            n191 = Enqueue Element(queue=w320, element=w319) -> (error out=w318:errorcluster)  [unwired: 2 in, 2 out]
          }
        }
        n192 = Merge Errors(w298, w305) -> (w307:errorcluster)
      }
      frame "Read TDMS" {
        n193 = call <vilib>:"Is Path and Not Empty.vi"("path"="tdms path") -> ("Is Path and Not Empty?"=w334:bool)  [unwired: 4 in]
        n194 = case shown="False" w334 {
          tunnel: "tdms path" -> [_ w363]
          tunnel: w333 -> [w338 w345]
          tunnel: [w337 w351] -> w328
          tunnel: [w336 w342] -> w331
          tunnel: w330 -> [w336 _]
          frame False {
            w341 = T1 {"data"=variant, "state"=enum."Initialize 1"}  # Cluster
            w340 = state."Config file Error"  # state
            n195 = Bundle By Name(cluster=w341, "state"=w340) -> (w339:T1)
            n196 = Enqueue Element At Opposite End(queue=w338, element=w339) -> (error out=w337:errorcluster)  [unwired: 2 in, 2 out]
          }
          frame True {
            w344 = T1 {"data"=variant, "state"=enum."Initialize 1"}  # Cluster
            w357 = "Version History" ("group name in (Untitled)")
            n197 = TDMS Open(11:w363) -> (0:w362:errorcluster, 3:w361:refnum<k34>)  [unwired: 6 in]
            n198 = TDMS List Contents(4:w362, 6:w357, 7:w361) -> (1:w354:string[], 3:w356:refnum<k34>)  [unwired: 2 out]
            n199 = Array Size(array=w354) -> (size(s)=w353:i32)
            n200 = Reverse 1D Array(array=w354) -> (reversed array=w360:string[])
            n201 = Index Array(array=w360, index=0) -> (element=w358:string)
            n202 = TDMS Read(0:w356, 5:w357, 7:w358, 12:string[] []) -> (4:w342:refnum<k34>, 10:w352:string[])  [unwired: 4 in, 4 out]
            n203 = case shown="1" w353 {
              tunnel: w352 -> [w364 w366]
              tunnel: [w364 w365] -> w349
              frame 2, Default {
              }
              frame 1 {
                n204 = for {
                  tunnel: w366 -> [_] mode=indexing
                  tunnel: ["no records!"] -> w365 mode=indexing
                }
              }
            }
            n205 = Array Size(array=w349) -> (size(s)=w350:i32)
            n206 = Bundle(w349, w350) -> (w348:cluster{string[], i32})  [unwired: 1 in]
            n207 = To Variant(anything=w348) -> (Variant=w347:variant)
            n208 = Bundle By Name(cluster=w344, "state"=state."Update Current Versions", "data"=w347) -> (w343:T1)
            n209 = Enqueue Element(queue=w345, element=w343) -> (error out=w351:errorcluster)  [unwired: 2 in, 2 out]
          }
        }
        n210 = Merge Errors(w332, w328) -> (w335:errorcluster)
      }
      frame "Update Comp Names" {
        w374 = T1 {"data"=variant, "state"=enum."Initialize 1"}  # Cluster
        w373 = state."Idle"  # state
        n211 = Variant To Data(type=cluster{"all rows":string[][], i32[]} {"all rows"=[], []} ("output cluster"), Variant=w384) -> (data=w382:cluster{"all rows":string[][], i32[]})  [unwired: 1 in, 1 out]
        n212 = Unbundle By Name(w371) -> ("Names"=w370:refnum<vi>[])
        n213 = Unbundle(w382) -> ("all rows"=w380:string[][])  [unwired: 1 out]
        n214 = Index Array(array=w380, index (col)=0 ("disabled index (col)")) -> (element=w378:string[])  [unwired: 1 in]
        n215 = for {
          shift-right: [w387] -> w377
          shift-left: w381 -> [w390]
          tunnel: w378 -> [w388] mode=indexing
          tunnel: w370 -> [w385] mode=indexing
          n216 = property class="Str"(reference=w385, error in=w390, "Visible"=TRUE) -> (reference out=w386:refnum<vi>, error out=w389:errorcluster)
          n217 = property class="Str"(reference=w386, error in=w389, "Value"=w388) -> (error out=w387:errorcluster)  [unwired: 1 out]
        }
        n218 = Bundle By Name(cluster=w374, "state"=w373) -> (w372:T1)
        n219 = Enqueue Element(queue=w376, element=w372, error in (no error)=w377) -> (error out=w375:errorcluster)  [unwired: 1 in, 2 out]
      }
      frame "Update Current Versions" {
        w392 = state."Check current versions"  # state
        w403 = T1 {"data"=variant, "state"=enum."Initialize 1"}  # Cluster
        n220 = Unbundle By Name(w398) -> ("Current Versions"=w397:refnum<vi>[], "New Versions"=w396:refnum<vi>[], "Names"=w394:refnum<vi>[])
        n221 = Variant To Data(type=cluster{string[], i32} {[], 0} ("output cluster"), Variant=w407) -> (data=w408:cluster{string[], i32})  [unwired: 1 in, 1 out]
        n222 = Unbundle(w408) -> (w405:string[])  [unwired: 1 out]
        n223 = while {
          shift-right: [w423] -> w401
          shift-left: w404 -> [w416]
          tunnel: w405 -> [w427] mode=indexing
          tunnel: w397 -> [w425] mode=indexing
          tunnel: w396 -> [w422] mode=indexing
          tunnel: w394 -> [w413]
          i -> [w410]
          stop <- w414 continue-if-true
          w421 = TRUE ("Visible")
          n224 = Add(x=1.0, y=w410) -> (x+y=w412:dbl)
          n225 = property class="Str"(reference=w425, error in=w416, "Visible"=w421) -> (reference out=w426:refnum<vi>, error out=w428:errorcluster)
          n226 = property class="Str"(reference=w422, error in=w416, "Visible"=w421) -> (reference out=w420:refnum<vi>, error out=w419:errorcluster)
          n227 = Index Array(array=w413, index=w412) -> (element=w409:refnum<vi>)
          n228 = property class="Str"(reference=w426, error in=w428, "Value"=w427) -> (error out=w424:errorcluster)  [unwired: 1 out]
          n229 = property class="Str"(reference=w420, error in=w419, "Value"="") -> (error out=w418:errorcluster)  [unwired: 1 out]
          n230 = property class="Str"(reference=w409, error in=w416) -> (error out=w415:errorcluster, "Visible"=w414:bool)  [unwired: 1 out]
          n231 = Merge Errors(w424, w418, w415) -> (w423:errorcluster)
        }
        n232 = Bundle By Name(cluster=w403, "state"=w392) -> (w402:T1)
        n233 = Enqueue Element(queue=w400, element=w402, error in (no error)=w401) -> (error out=w399:errorcluster)  [unwired: 1 in, 2 out]
      }
      frame "Make new configuration" {
        w438 = T1 {"data"=variant, "state"=enum."Initialize 1"}  # Cluster
        n234 = Unbundle By Name(w446) -> ("New Versions"=w445:refnum<vi>[], "Current Versions"=w444:refnum<vi>[])
        n235 = Initialize Array "Initialize Array"("", w440) -> (w441:string[])
        n236 = for {
          N: w440 -> [_]
          tunnel: w445 -> [w462] mode=indexing
          tunnel: w444 -> [w468] mode=indexing
          shift-right: [w452] -> w437
          shift-left: w443 -> [w461]
          shift-right: [w460] -> w439
          shift-left: w441 -> [w464]
          shift-right: [w454] -> w432
          shift-left: 0 -> [w455]
          i -> [w463]
          n237 = property class="Str"(reference=w468, error in=w461) -> (error out=w458:errorcluster, "Value"=w467:string)  [unwired: 1 out]
          n238 = property class="Str"(reference=w462, error in=w461) -> (reference out=w456:refnum<vi>, error out=w459:errorcluster, "Value"=w465:string)
          n239 = Merge Errors(w459, w458) -> (w450:errorcluster)
          n240 = Empty String/Path?(string/path=w465) -> (empty?=w466:bool)
          n241 = case shown="False" w466 {
            tunnel: w467 -> [_ w478]
            tunnel: [w475 w478] -> w457
            tunnel: w465 -> [w475 _]
            tunnel: w456 -> [w474 _]
            tunnel: w455 -> [w472 w477]
            tunnel: [w471 w477] -> w454
            tunnel: [w470 w476] -> w451
            tunnel: w450 -> [w469 w476]
            frame False {
              # "new version"
              n242 = Increment(x=w472) -> (x+1=w471:i32)
              n243 = property class="Str"(reference=w474, error in=w469, "Text.TextColor"=u32 16714752) -> (error out=w470:errorcluster)  [unwired: 1 out]
            }
            frame True {
              # "no new version"
            }
          }
          n244 = property class="Str"(reference=w456, error in=w450, "Value"=w457) -> (error out=w453:errorcluster)  [unwired: 1 out]
          n245 = Replace Array Subset(array=w464, new element=w457, index=w463) -> (w460:string[])
          n246 = Merge Errors(w453, w451) -> (w452:errorcluster)
        }
        n247 = Equal To 0?(x=w432) -> (x = 0?=w431:bool)
        n248 = case shown="True" w431 {
          tunnel: [w448 w449] -> w429
          frame False {
            w448 = state."Register Change"  # state
            # "There is at least one new version"
          }
          frame True {
            w449 = state."No New Update"  # state
            # "No New Updates"
          }
        }
        n249 = To Variant(anything=w439) -> (Variant=w430:variant)
        n250 = Bundle By Name(cluster=w438, "state"=w429, "data"=w430) -> (w435:T1)
        n251 = Enqueue Element(queue=w434, element=w435, error in (no error)=w437) -> (error out=w436:errorcluster)  [unwired: 1 in, 2 out]
      }
      frame "Register Change" {
        n252 = Variant To Data(error in=w490, type=string[] [], Variant=w491) -> (data=w488:string[], error out=w483:errorcluster)
        n253 = call "Confirm changes"("error in (no error)"=w483) -> ("Sign with your name"=w480:string, "Confirm"=w481:bool, "error out"=w482:errorcluster)  [unwired: 16 in]
        n254 = case shown="True" w481 {
          tunnel: w487 -> [_ w503]
          tunnel: w482 -> [w493 w505]
          tunnel: w488 -> [_ w513]
          tunnel: [w492 w508] -> w486
          tunnel: w485 -> [w498 w509]
          tunnel: ["M400: The configuration was rejected." ("F button name (\"Cancel\")") "M300: The configuration was successfully registered." ("F button name (\"Cancel\")")] -> w484
          tunnel: w480 -> [_ w500]
          frame False {
            w497 = T1 {"data"=variant, "state"=enum."Initialize 1"}  # Cluster
            w496 = state."Initialize 2"  # state
            n255 = Bundle By Name(cluster=w497, "state"=w496) -> (w495:T1)
            n256 = Enqueue Element(queue=w498, element=w495, error in (no error)=w493) -> (error out=w492:errorcluster)  [unwired: 1 in, 2 out]
          }
          frame True {
            w512 = T1 {"data"=variant, "state"=enum."Initialize 1"}  # Cluster
            w511 = state."Idle"  # state
            n257 = Build Array(w500) -> (w499:string[])
            n258 = Get Date/Time In Seconds() -> (seconds since 1Jan1904=w514:timestamp)
            n259 = Format Date/Time String(time format string (%c)="Date: %Y-%b-%d    Time: %H:%M:%S", seconds (now)=w514) -> (date/time string=w501:string)  [unwired: 1 in]
            n260 = TDMS Write(0:w503, 5:"Reporter" ("group name in (Untitled)"), 7:w501, 9:w499, 11:w505) -> (15:w504:errorcluster)  [unwired: 1 in, 3 out]
            n261 = TDMS Write(0:w503, 5:"Version History" ("group name in (Untitled)"), 7:w501, 9:w513, 11:w504) -> (15:w507:errorcluster)  [unwired: 1 in, 3 out]
            n262 = Bundle By Name(cluster=w512, "state"=w511) -> (w510:T1)
            n263 = Enqueue Element(queue=w509, element=w510, error in (no error)=w507) -> (error out=w508:errorcluster)  [unwired: 1 in, 2 out]
          }
        }
        "Status bar" <- w484
      }
      frame "View Registry" {
        w522 = T1 {"data"=variant, "state"=enum."Initialize 1"}  # Cluster
        w521 = state."Idle"  # state
        n264 = property on="tdms path" class="Path"(error in=w525) -> (error out=w523:errorcluster, "Value"=w524:path)  [unwired: 1 in, 1 out]
        n265 = call <vilib>:"TDMS - File Viewer.vi"("error in (no error)"=w523, "file path"=w524) -> ("error out"=w518:errorcluster)  [unwired: 4 in, 1 out]
        n266 = Bundle By Name(cluster=w522, "state"=w521) -> (w519:T1)
        n267 = Enqueue Element(queue=w520, element=w519, error in (no error)=w518) -> (error out=w517:errorcluster)  [unwired: 1 in, 2 out]
      }
      frame "Add Comment" {
        n268 = call "Comment"("error in (no error)"=w532) -> ("Name"=w531:string, "Comment"=w537:string, "Add"=w536:bool, "error out"=w534:errorcluster)  [unwired: 15 in]
        n269 = TDMS List Contents(4:w532, 6:"Version History" ("group name in (Untitled)"), 7:w542) -> (0:w533:errorcluster, 1:w543:string[], 3:w544:refnum<k34>)  [unwired: 1 out]
        n270 = Reverse 1D Array(array=w543) -> (reversed array=w546:string[])
        n271 = Index Array(array=w546, index=0) -> (element=w539:string)
        n272 = Merge Errors(w534, w533) -> (w535:errorcluster)
        n273 = case shown="True" w536 {
          tunnel: w544 -> [w550 w559]
          tunnel: w535 -> [w549 w558]
          tunnel: "Comment" ("group name in (Untitled)") -> [_ w557]
          tunnel: w539 -> [_ w555]
          tunnel: [w550 w556] -> w538
          tunnel: w537 -> [_ w554]
          tunnel: [w549 w552] -> w530
          tunnel: w531 -> [_ w551]
          frame False {
          }
          frame True {
            n274 = Build Array(w551, w554) -> (w553:string[])
            n275 = TDMS Write(0:w559, 5:w557, 7:w555, 9:w553, 11:w558) -> (4:w556:refnum<k34>, 15:w552:errorcluster)  [unwired: 1 in, 2 out]
          }
        }
        n276 = property on="Status bar" class="Str"(error in=w530, "Value"="M500: Comment was successfully added to the latest entry." ("Status bar")) -> (error out=w528:errorcluster)  [unwired: 1 in, 1 out]
      }
      frame "No New Update" {
        w565 = T1 {"data"=variant, "state"=enum."Initialize 1"}  # Cluster
        w560 = state."Initialize 2"  # state
        n277 = flat-sequence {
          tunnel: w566 -> [w572]
          tunnel: [w572] -> w564
          tunnel: [w569] -> _
          frame #0 {
            n278 = One Button Dialog(message="There is no new updates. To register a new configuration, you need at least one new version.\nThe page will be reinitialized with the latest configuration.", button name ("OK")="OK") -> (true=w569:bool)
          }
        }
        n279 = Bundle By Name(cluster=w565, "state"=w560) -> (w561:T1)
        n280 = Enqueue Element(queue=w563, element=w561, error in (no error)=w564) -> (error out=w562:errorcluster)  [unwired: 1 in, 2 out]
      }
      frame "Check current versions" {
        n281 = Unbundle By Name(w576) -> ("Current Versions"=w575:refnum<vi>[])
        n282 = for {
          N: w577 -> [_]
          tunnel: w575 -> [w586] mode=indexing
          shift-right: [w581] -> w573
          shift-left: w574 -> [w585]
          n283 = property class="Str"(reference=w586, error in=w585) -> (reference out=w580:refnum<vi>, error out=w582:errorcluster, "Value"=w584:string)
          n284 = Empty String/Path?(string/path=w584) -> (empty?=w583:bool)
          n285 = case shown="True" w583 {
            tunnel: w582 -> [w587 _]
            tunnel: [w587 w590] -> w581
            tunnel: w580 -> [_ w589]
            frame False {
              # "version exits"
            }
            frame True {
              n286 = property class="Str"(reference=w589, "Value"="no records!") -> (error out=w590:errorcluster)  [unwired: 1 in, 1 out]
            }
          }
        }
      }
      frame "Config file Error" {
        n287 = One Button Dialog(message="Error in (txt or tdms) file path.\nEither Not A Path or Path is Empty.", button name ("OK")="Close Application") -> (true=w596:bool)
        n288 = case shown="True" w596 {
          tunnel: w591 -> [_ w599]
          frame False {
          }
          frame True {
            w600 = T1 {"data"=variant, "state"=enum."Initialize 1"}  # Cluster
            w601 = state."Close"  # state
            n289 = Bundle By Name(cluster=w600, "state"=w601) -> (w598:T1)
            n290 = Enqueue Element At Opposite End(queue=w599, element=w598) -> ()  [unwired: 2 in, 3 out]
          }
        }
      }
      frame "Write ini file" {
        w610 = T1 {"data"=variant, "state"=enum."Initialize 1"}  # Cluster
        w611 = state."Close"  # state
        w621 = "Path" ("section")
        n291 = Current VI's Path() -> (path=w603:path)
        n292 = Bundle By Name(cluster=w610, "state"=w611) -> (w605:T1)
        n293 = disable-structure shown="RUN_TIME_ENGINE==True" {
          disable-tunnel: w603 -> [w633 w637]
          disable-tunnel: [w632 w634] -> w602
          frame condition #0 (active) {
            n294 = Strip Path(path=w633) -> (stripped path=w632:path)  [unwired: 1 out]
          }
          frame condition #1 {
            n295 = Strip Path(path=w637) -> (stripped path=w636:path)  [unwired: 1 out]
            n296 = Strip Path(path=w636) -> (stripped path=w635:path)  [unwired: 1 out]
            n297 = Strip Path(path=w635) -> (stripped path=w634:path)  [unwired: 1 out]
          }
        }
        n298 = property on="Config Path" class="Path"(error in=w607) -> (error out=w616:errorcluster, "Value"=w615:path)  [unwired: 1 in, 1 out]
        n299 = Enqueue Element(queue=w609, element=w605, error in (no error)=w607) -> (queue out=w608:refnum<queue>, error out=w606:errorcluster)  [unwired: 1 in, 1 out]
        n300 = Build Path(base path=w602, name or relative path=path "Register Change.ini") -> (appended path=w628:path)
        n301 = call <vilib>:"Open Config Data.vi"("error in (no error)"=w607, "create file if necessary (T)"=FALSE, "configuration file path"=w628) -> ("error out"=w626:errorcluster, "refnum"=w627:T6)  [unwired: 6 in, 1 out]
        n302 = call-poly <vilib>:"Write Key.vi"("section"=w621, "error in (no error)"=w626, "value"=w615, "key"="txt config file", "refnum"=w627) -> ("error out"=w624:errorcluster, "refnum out"=w623:T6)  [unwired: 4 in, 1 out]
        n303 = property on="tdms path" class="Path"(error in=w616) -> (error out=w613:errorcluster, "Value"=w614:path)  [unwired: 1 in, 1 out]
        n304 = call-poly <vilib>:"Write Key.vi"("section"=w621, "error in (no error)"=w624, "value"=w614, "key"="tdms file", "refnum"=w623) -> ("error out"=w618:errorcluster, "refnum out"=w617:T6)  [unwired: 4 in, 1 out]
        n305 = call <vilib>:"Close Config Data.vi"("error in (no error)"=w618, "refnum"=w617) -> ("error out"=w619:errorcluster)  [unwired: 8 in, 1 out]
        n306 = Merge Errors(w619, w613) -> (w604:errorcluster)
        n307 = Merge Errors(w606, w604) -> (w612:errorcluster)
      }
      frame "Close" {
        n308 = control-ref of="Run"() -> (w644:refnum<vi>)
        n309 = property class="Bool"(reference=w644, error in=w642, "DisabledEnum"=T5."Enabled" ("Disabled")) -> (error out=w641:errorcluster)  [unwired: 1 out]
        n310 = Release Queue(queue=w652, error in (no error)=w642) -> (error out=w651:errorcluster)  [unwired: 1 in, 2 out]
        n311 = TDMS Close(8:w642, 11:w645) -> (0:w646:errorcluster)  [unwired: 1 out]
        n312 = property on="Status bar" class="Str"(error in=w641, "Value"="M700: Application ended." ("Status bar")) -> (error out=w640:errorcluster)  [unwired: 1 in, 1 out]
        n313 = Merge Errors(w651, w646, w640) -> (w650:errorcluster)
        n314 = disable-structure shown="Default" {
          disable-tunnel: w650 -> [w654 w656]
          disable-tunnel: [w654 w656] -> w649
          disable-tunnel: TRUE ("quit? (T)") -> [w653 w655]
          frame condition #0 (active) {
            n315 = Stop(stop? (T)=w653) -> ()
          }
          frame condition #1 {
            n316 = Quit LabVIEW(quit? (T)=w655) -> ()
          }
        }
      }
    }
  }
  n317 = while {
    tunnel: w87 -> [w658]
    stop <- w657 stop-if-true
    n318 = Wait (ms)(milliseconds to wait=u32 50) -> ()  [unwired: 1 out]
    n319 = event shown="[7] \"Help Button\": Value Change" {
      selector: _ -> [_ _ _ _ _ _ _ _]
      dyn-events: _ -> [_ _ _ _ _ _ _ _]
      timeout: _ -> [_ _ _ _ _ _ _ _]
      tunnel: w658 -> [_ w662 w670 w674 w682 w685 w689 _]
      tunnel: [_ TRUE _ _ _ _ _ _] -> w657
      tunnel: [_ w660 w666 w673 w678 w683 w688 w695] -> _
      event Timeout {
        n320 = event-data() -> ()  [unwired: 1 in, 2 out]
      }
      event "Exit": Value Change {
        w665 = T1 {"data"=variant, "state"=enum."Initialize 1"}  # Cluster
        w664 = state."Write ini file"  # state
        n321 = event-data() -> ()  [unwired: 1 in, 6 out]
        n322 = Bundle By Name(cluster=w665, "state"=w664) -> (w663:T1)
        n323 = Enqueue Element At Opposite End(queue=w662, element=w663) -> (error out=w660:errorcluster)  [unwired: 2 in, 2 out]
      }
      event "Register change": Value Change {
        w672 = T1 {"data"=variant, "state"=enum."Initialize 1"}  # Cluster
        w669 = state."Make new configuration"  # state
        n324 = event-data() -> ()  [unwired: 1 in, 6 out]
        n325 = Bundle By Name(cluster=w672, "state"=w669) -> (w671:T1)
        n326 = Enqueue Element(queue=w670, element=w671) -> (error out=w667:errorcluster)  [unwired: 2 in, 2 out]
        n327 = property on="Register change" class="Bool"(error in=w667, "DisabledEnum"=T5."Disabled and Grayed Out" ("Disabled")) -> (error out=w666:errorcluster)  [unwired: 1 in, 1 out]
      }
      event "Initialize": Value Change {
        w677 = T1 {"data"=variant, "state"=enum."Initialize 1"}  # Cluster
        w675 = state."Initialize 2"  # state
        n328 = event-data() -> ()  [unwired: 1 in, 6 out]
        n329 = Bundle By Name(cluster=w677, "state"=w675) -> (w676:T1)
        n330 = Enqueue Element(queue=w674, element=w676) -> (error out=w673:errorcluster)  [unwired: 2 in, 2 out]
      }
      event "Add comment": Value Change {
        w680 = T1 {"data"=variant, "state"=enum."Initialize 1"}  # Cluster
        w679 = state."Add Comment"  # state
        n331 = event-data() -> ()  [unwired: 1 in, 6 out]
        n332 = Bundle By Name(cluster=w680, "state"=w679) -> (w681:T1)
        n333 = Enqueue Element(queue=w682, element=w681) -> (error out=w678:errorcluster)  [unwired: 2 in, 2 out]
      }
      event "Run": Value Change {
        w687 = T1 {"data"=variant, "state"=enum."Initialize 1"}  # Cluster
        w686 = state."Initialize 1"  # state
        n334 = event-data() -> ()  [unwired: 1 in, 6 out]
        n335 = Bundle By Name(cluster=w687, "state"=w686) -> (w684:T1)
        n336 = Enqueue Element(queue=w685, element=w684) -> (error out=w683:errorcluster)  [unwired: 2 in, 2 out]
      }
      event "View": Value Change {
        w692 = T1 {"data"=variant, "state"=enum."Initialize 1"}  # Cluster
        w691 = state."View Registry"  # state
        n337 = event-data() -> ()  [unwired: 1 in, 6 out]
        n338 = Bundle By Name(cluster=w692, "state"=w691) -> (w690:T1)
        n339 = Enqueue Element(queue=w689, element=w690) -> (error out=w688:errorcluster)  [unwired: 2 in, 2 out]
      }
      event "Help Button": Value Change {
        n340 = event-data() -> ()  [unwired: 1 in, 6 out]
        n341 = Current VI's Path() -> (path=w694:path)
        n342 = disable-structure shown="Default" {
          disable-tunnel: w694 -> [w700 w706]
          disable-tunnel: [w697 w702] -> w693
          frame condition #0 (active) {
            n343 = Strip Path(path=w700) -> (stripped path=w699:path)  [unwired: 1 out]
            n344 = Build Path(base path=w699, name or relative path=path "../documentation/help.mht") -> (appended path=w697:path)
          }
          frame condition #1 {
            n345 = Strip Path(path=w706) -> (stripped path=w705:path)  [unwired: 1 out]
            n346 = Strip Path(path=w705) -> (stripped path=w704:path)  [unwired: 1 out]
            n347 = Strip Path(path=w704) -> (stripped path=w701:path)  [unwired: 1 out]
            n348 = Build Path(base path=w701, name or relative path=path "data/help.mht") -> (appended path=w702:path)
          }
        }
        n349 = Control Online Help(2:w693, 4:enum16{"Contents", "Key", "Close"}."Contents" ("Operation")) -> (0:w695:errorcluster)  [unwired: 2 in]
      }
    }
  }
  n350 = Release Queue(queue=w2, error in (no error)=w3) -> (error out=w1:errorcluster)  [unwired: 1 in, 2 out]
  n351 = call <vilib>:"Simple Error Handler.vi"("error in (no error)"=w1) -> ()  [unwired: 4 in, 5 out]
